vi "NF LI56xx sub set sig.vi"(7 "Type":string, 8 "error in":errorcluster caption="error in (no error)" {"code" format="%.0x"}, 10 "Input":T1, 11 "VISA resource name":refnum<visa-resource-name>) -> (0 "error out":errorcluster {"code" format="%.0x"}, 2 "change input type":bool, 3 "VISA resource name copy":refnum<visa-resource-name>)   [LabVIEW 2019]
doc: "set input signal related parameters"
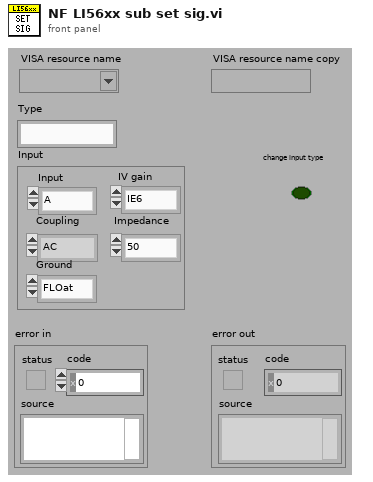
[diagram p1: front panel]
types:
  T1 = cluster{" Input":enum16{"A", "AB", "C", "I", "HF"}, "Coupling":enum16{"AC", "DC"}, "Ground":enum16{"FLOat", "GROund"}, "IV gain":enum16{"IE6", "IE8"}, "Impedance":enum16{"50", "1E6"}}
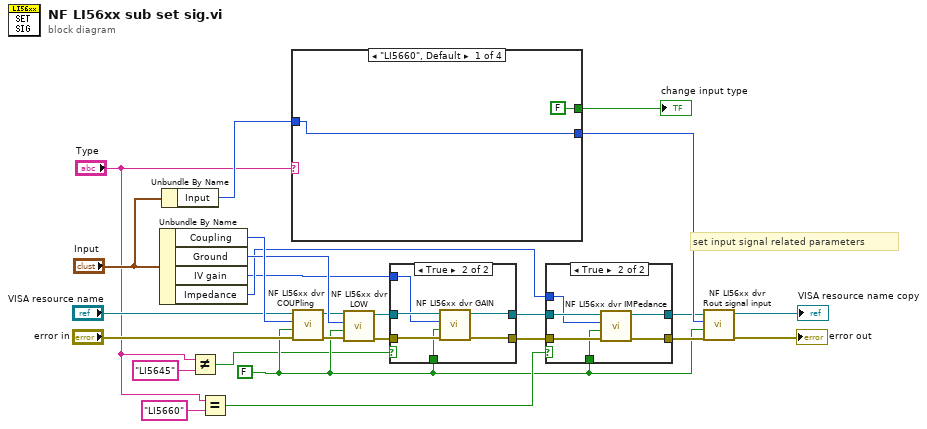
[diagram p0: block diagram]
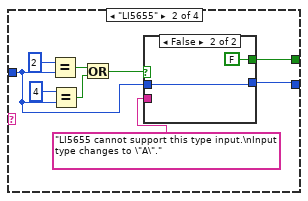
[diagram p4: hidden frame]
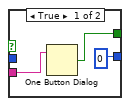
[diagram p5: hidden frame]
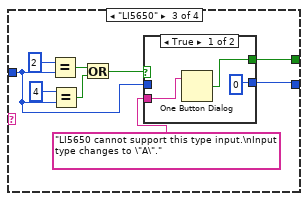
[diagram p6: hidden frame]
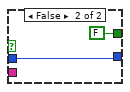
[diagram p7: hidden frame]
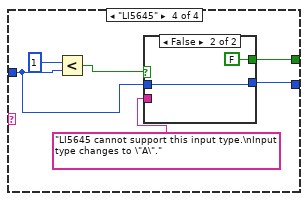
[diagram p8: hidden frame]
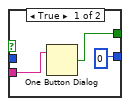
[diagram p9: hidden frame]
diagram:
  w8 = FALSE ("Read(F)")
  # "set input signal related parameters"
  n1 = Unbundle By Name("Input") -> ("Coupling"=w26:enum16{"AC", "DC"}, "Ground"=w25:enum16{"FLOat", "GROund"}, "IV gain"=w5:enum16{"IE6", "IE8"}, "Impedance"=w11:enum16{"50", "1E6"})
  n2 = Unbundle By Name("Input") -> ("Input"=w16:enum16{"A", "AB", "C", "I", "HF"})
  n3 = Not Equal?(x="Type", y="LI5645") -> (x != y?=w2:bool)
  n4 = Equal?(x="Type", y="LI5660") -> (x = y?=w12:bool)
  n5 = case shown="\"LI5660\", Default" "Type" {
    tunnel: [w28 w37 w51 w62] -> w17
    tunnel: w16 -> [w28 w30 w44 w59]
    tunnel: [FALSE ("true") w29 w43 w57] -> w1
    frame "LI5660", Default {
    }
    frame "LI5655" {
      n6 = Equal?(x=2 ("t"), y=w30) -> (x = y?=w33:bool)
      n7 = Equal?(x=4 ("t"), y=w30) -> (x = y?=w32:bool)
      n8 = Or(x=w33, y=w32) -> (x .or. y?=w31:bool)
      n9 = case shown="False" w31 {
        tunnel: "LI5655 cannot support this type input.\nInput type changes to \"A\"." -> [w40 _]
        tunnel: [0 ("t") w42] -> w37
        tunnel: w30 -> [_ w42]
        tunnel: [w38 FALSE ("true")] -> w29
        frame True {
          n10 = One Button Dialog(message=w40) -> (true=w38:bool)  [unwired: 1 in]
        }
        frame False {
        }
      }
    }
    frame "LI5650" {
      n11 = Equal?(x=2 ("t"), y=w44) -> (x = y?=w47:bool)
      n12 = Equal?(x=4 ("t"), y=w44) -> (x = y?=w46:bool)
      n13 = Or(x=w47, y=w46) -> (x .or. y?=w45:bool)
      n14 = case shown="True" w45 {
        tunnel: "LI5650 cannot support this type input.\nInput type changes to \"A\"." -> [w54 _]
        tunnel: [0 ("t") w56] -> w51
        tunnel: w44 -> [_ w56]
        tunnel: [w52 FALSE ("true")] -> w43
        frame True {
          n15 = One Button Dialog(message=w54) -> (true=w52:bool)  [unwired: 1 in]
        }
        frame False {
        }
      }
    }
    frame "LI5645" {
      n16 = Less?(x=1 ("t"), y=w59) -> (x < y?=w58:bool)
      n17 = case shown="False" w58 {
        tunnel: "LI5645 cannot support this input type.\nInput type changes to \"A\"." -> [w65 _]
        tunnel: [0 ("t") w67] -> w62
        tunnel: w59 -> [_ w67]
        tunnel: [w63 FALSE ("true")] -> w57
        frame True {
          n18 = One Button Dialog(message=w65) -> (true=w63:bool)  [unwired: 1 in]
        }
        frame False {
        }
      }
    }
  }
  "change input type" <- w1
  n19 = call "NF LI56xx dvr COUPling.vi"("error in"="error in", "Read(F)"=w8, "set coupling"=w26, "VISA resource name"="VISA resource name") -> ("error out"=w23:errorcluster, "VISA resource name copy"=w24:refnum<visa-resource-name>)  [unwired: 5 in, 1 out]
  n20 = call "NF LI56xx dvr LOW.vi"("error in"=w23, "Read(F)"=w8, "set grounding"=w25, "VISA resource name"=w24) -> ("error out"=w9:errorcluster, "VISA resource name copy"=w10:refnum<visa-resource-name>)  [unwired: 5 in, 1 out]
  n21 = case shown="True" w2 {
    tunnel: w10 -> [w69 w74]
    tunnel: w9 -> [w68 w73]
    tunnel: [w69 w75] -> w6
    tunnel: [w68 w72] -> w7
    tunnel: w8 -> [_ w71]
    tunnel: w5 -> [_ w70]
    frame False {
    }
    frame True {
      n22 = call "NF LI56xx dvr GAIN.vi"("error in"=w73, "Read(F)"=w71, "set IV gain"=w70, "VISA resource name"=w74) -> ("error out"=w72:errorcluster, "VISA resource name copy"=w75:refnum<visa-resource-name>)  [unwired: 5 in, 1 out]
    }
  }
  n23 = case shown="True" w12 {
    tunnel: w6 -> [w77 w83]
    tunnel: w7 -> [w76 w82]
    tunnel: [w77 w81] -> w15
    tunnel: [w76 w80] -> w14
    tunnel: w11 -> [_ w79]
    tunnel: w8 -> [_ w78]
    frame False {
    }
    frame True {
      n24 = call "NF LI56xx dvr IMPedance.vi"("error in"=w82, "Read(F)"=w78, "set input impedance"=w79, "VISA resource name"=w83) -> ("error out"=w80:errorcluster, "VISA resource name copy"=w81:refnum<visa-resource-name>)  [unwired: 5 in, 1 out]
    }
  }
  n25 = call "NF LI56xx dvr Rout signal input.vi"("error in"=w14, "Read(F)"=w8, "set signal input"=w17, "VISA resource name"=w15) -> ("error out"=→"error out":errorcluster, "VISA resource name copy"=→"VISA resource name copy":refnum<visa-resource-name>)  [unwired: 5 in, 1 out]
